vi "Read Events.vi"(8 "error in (no error)":errorcluster, 11 "TestApplication in":refnum<class "TestApplication.lvclass">) -> (0 "error out":errorcluster, 2 "Events":T1, 3 "TestApplication out":refnum<class "TestApplication.lvclass">)   [LabVIEW 2022 SP3, in "Demo.lvlib" / "TestApplication.lvclass"]
uses:
  TestApplication.lvclass
  _Events.ctl
  TestApplication.lvclass/TestApplication.ctl
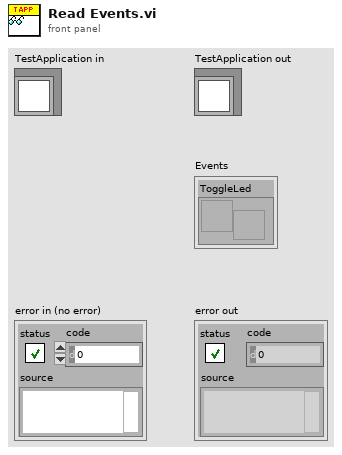
[diagram p1: front panel]
types:
  T1 = typedef "Demo.lvlib/TestApplication.lvclass/_Events.ctl" = cluster{"ToggleLed":refnum<user-event>}
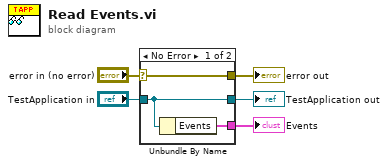
[diagram p0: block diagram]
diagram:
  n1 = case shown="No Error" "error in (no error)" {
    selector: "error in (no error)" -> [w8 w9]
    tunnel: [w8 w9] -> w4
    tunnel: [w7 w10] -> w2
    tunnel: "TestApplication in" -> [w7 w10]
    tunnel: [w6 _] -> w1
    frame No Error {
      n2 = Unbundle By Name(w7) -> ("Events"=w6:T1)
    }
    frame Error {
    }
  }
  "error out" <- w4
  "TestApplication out" <- w2
  "Events" <- w1
